vi "1.8.vi"() -> ()   [LabVIEW 2017]
panel:
  out "led":bool
  in  "B":bool
  in  "A":bool
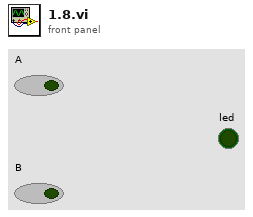
[diagram p1: front panel]
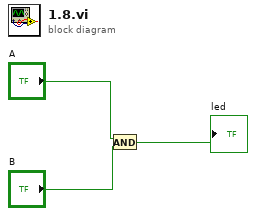
[diagram p0: block diagram]
diagram:
  n1 = And(x="A", y="B") -> (x .and. y?=→"led":bool)
